vi "MAX_Target.vi"(7 "Avaliable target xml files":path, 8 "Error in":errorcluster, 11 "Report Type":T1 items=["XML", "HTML", "Technical Support"]) -> (0 "error out":errorcluster)   [LabVIEW 2015]
uses:
  <vilib>/nisyscfg/Report Mode.ctl
  <vilib>/nisyscfg/Close (System).vi
  <vilib>/nisyscfg/nisyscfg.lvlib
panel:
  out "Number of target present":i32
  out "Detected Systems":string[](array[string])
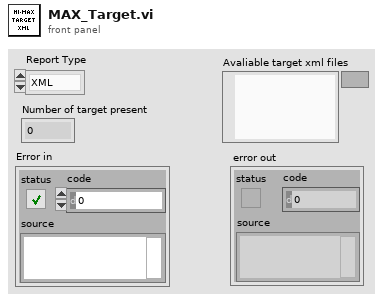
[diagram p1: front panel]
types:
  T1 = typedef "nisyscfg.lvlib/Report Mode.ctl" = i32
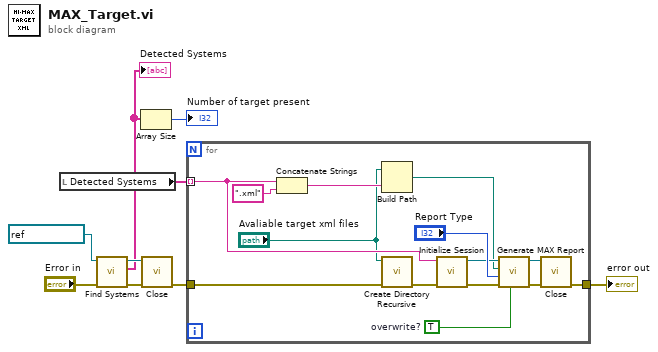
[diagram p0: block diagram]
diagram:
  n1 = local read "Detected Systems"() -> (w8:string[])
  n2 = call <vilib>:"Find Systems.vi"("error in (no error)"="Error in", "Session in (localhost)"=refnum<k21> "localhost") -> ("error out"=w4:errorcluster, "Detected Systems"=w2:string[], "Session out"=w5:refnum<k21>)  [unwired: 7 in]
  "Detected Systems" <- w2
  n3 = Array Size(array=w2) -> (size(s)=→"Number of target present":i32)
  n4 = call-poly <vilib>:"Close.vi"("error in (no error)"=w4, "Session in"=w5) -> ("error out"=w3:errorcluster)  [unwired: 9 in]
  n5 = for {
    tunnel: w8 -> [w12] mode=indexing
    tunnel: [w16] -> w9
    tunnel: w3 -> [w11]
    w23 = TRUE  # overwrite?
    n6 = Concatenate Strings(w12, ".xml" ("string")) -> (w14:string)
    n7 = Build Path(base path="Avaliable target xml files", name or relative path=w14) -> (appended path=w13:path)
    n8 = call <vilib>:"Create Directory Recursive.vi"("error in (no error)"=w11, "directory"="Avaliable target xml files") -> ("error out"=w17:errorcluster)  [unwired: 3 in, 2 out]
    n9 = call <vilib>:"Initialize Session.vi"("error in (no error)"=w17, "Target (localhost)"=w12) -> ("error out"=w21:errorcluster, "Session out"=w20:refnum<k21>)  [unwired: 8 in]
    n10 = call <vilib>:"Generate MAX Report.vi"("Overwrite (F)"=w23, "error in (no error)"=w21, "Report Type (XML)"="Report Type", "Output Filename"=w13, "Session in"=w20) -> ("error out"=w19:errorcluster, "Session out"=w18:refnum<k21>)  [unwired: 5 in]
    n11 = call-poly <vilib>:"Close.vi"("error in (no error)"=w19, "Session in"=w18) -> ("error out"=w16:errorcluster)  [unwired: 9 in]
  }
  "error out" <- w9
